vi "34970_CRISTALIZADOR_0 Module.vi"(5 "Agilent 34970A":bool=TRUE, 7 "Command":T1, 8 "error in (no error)":errorcluster, 10 "Canales":cluster{"CH PT100":string[], "CH TcK":string[]}={"CH PT100"=["201", "202", "205", "210"], "CH TcK"=["208"]}, 11 "VISA Agilent 34970A":refnum<visa-resource-name>="COM42") -> (0 "error out":errorcluster, 2 "TcK":dbl[](array[numeric]), 3 "PT100":dbl[](array[numeric]))   [LabVIEW 2017]
uses:
  34970_CRISTALIZADOR Module.ctl
  <instrlib>/Agilent 34970/Agilent 34970.lvlib
panel:
  # "Input Data"
  # "Output Data"
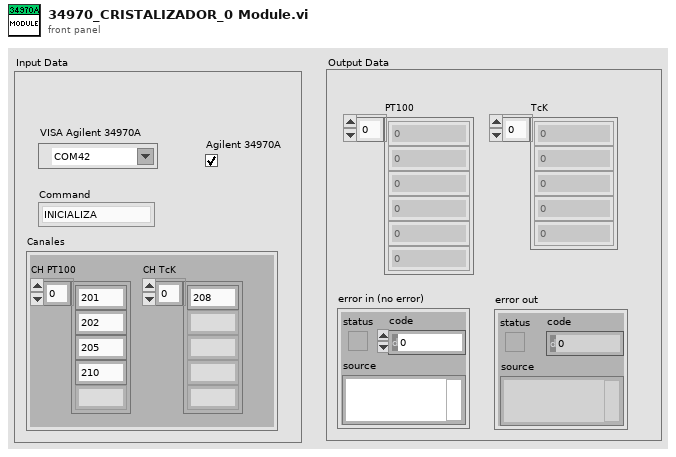
[diagram p1: front panel]
types:
  T1 = typedef "34970_CRISTALIZADOR Module.ctl" = enum16{"INICIALIZA", "CONFIGURA CANALES", "LECTURA PT100", "LECTURA TERMOPAR", "LECTURA VOLTAJE", "LECTURA CORRIENTE", "SHUTDOWN"}
  T2 = cluster{"Timeout Value (10000)":u32, "Baud Rate (57600)":enum16{"1200", "2400", "4800", "9600", "19200", "38400", "57600", "115200"}, "Flow Control (1:XON/XOFF)":enum16{"None", "XON / XOFF", "RTS / CTS", "DTR / DSR"}}
  T3 = enum16{"Thermocouple", "Thermistor", "RTD", "4-Wire RTD", "Default (Last)"}
  T4 = enum16{"B", "E", "J", "K", "N", "R", "S", "T", "Default (Last)"}
  T5 = enum16{"100 mV", "1 V", "10 V", "100 V", "300 V", "Auto", "Minimum", "Maximum"}
  T6 = enum16{"4 1/2", "5 1/2", "6 1/2", "Least", "Highest", "Default"}
  T7 = enum16{"10 mA", "100 mA", "1 A", "Auto", "Minimum", "Maximum"}
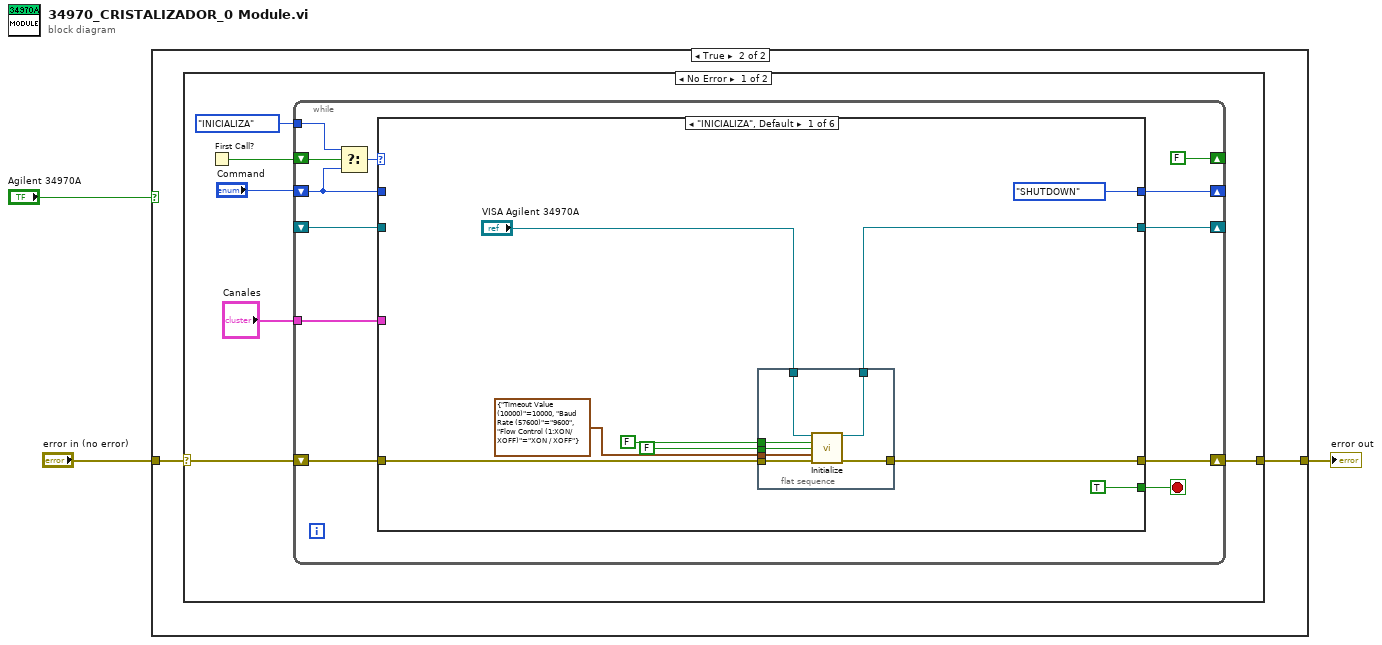
[diagram p0: block diagram]
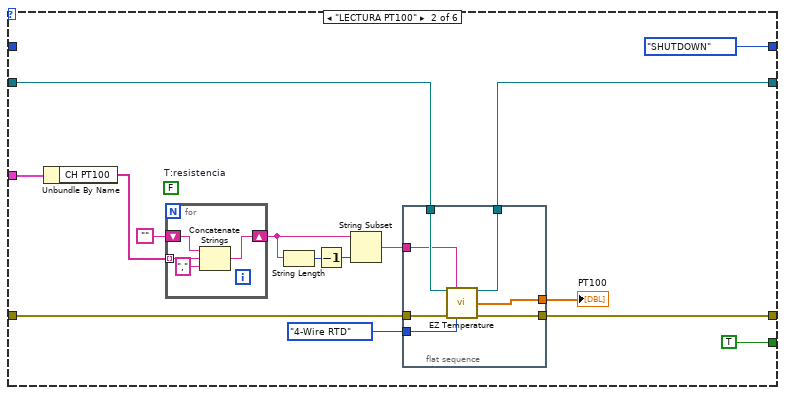
[diagram p3: hidden frame]
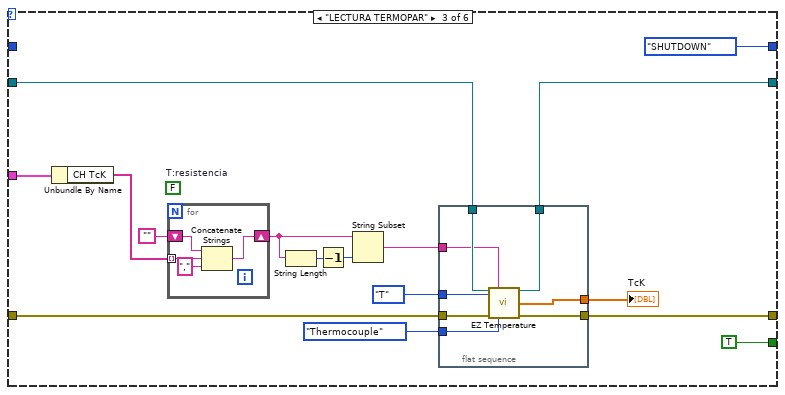
[diagram p4: hidden frame]
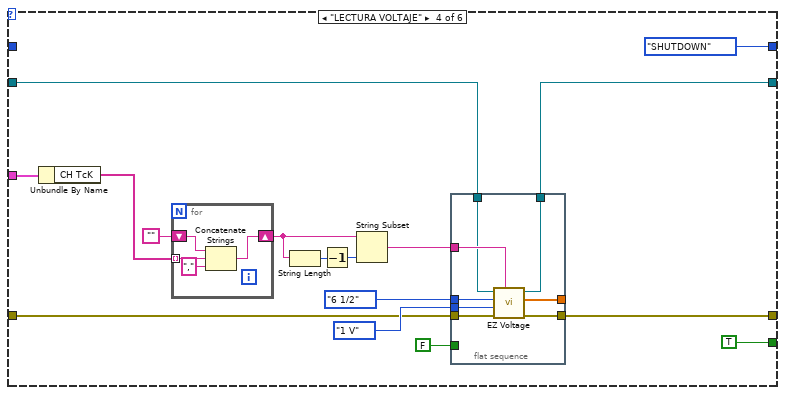
[diagram p5: hidden frame]
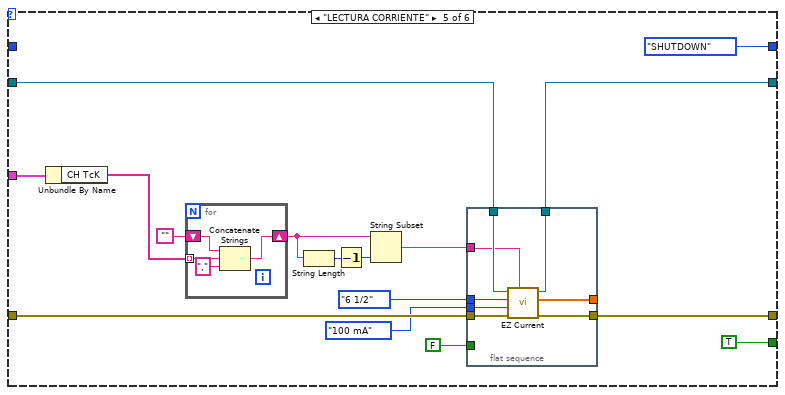
[diagram p6: hidden frame]
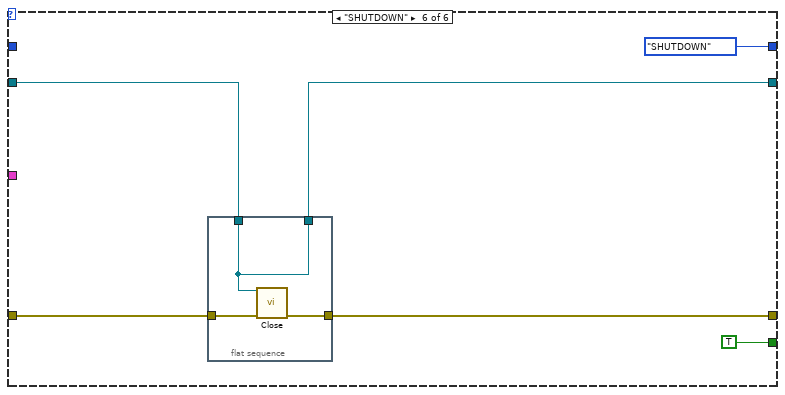
[diagram p7: hidden frame]
diagram:
  n1 = case shown="True" "Agilent 34970A" {
    tunnel: "error in (no error)" -> [w4 w6]
    tunnel: [w4 w5] -> w2
    frame False {
    }
    frame True {
      n2 = case shown="No Error" w6 {
        selector: w6 -> [w10 w160]
        tunnel: [w9 w160] -> w5
        frame No Error {
          n3 = First Call?() -> (First Call?: T/F=w12:bool)
          n4 = while {
            shift-right: [w18] -> _
            shift-left: "Command" -> [w19]
            shift-right: [w17] -> w9
            shift-left: w10 -> [w21]
            shift-right: [FALSE ("First Call?: T/F")] -> _
            shift-left: w12 -> [w24]
            tunnel: 34970_CRISTALIZADOR_Module."INICIALIZA" ("t") -> [w23]
            shift-right: [w15] -> _
            shift-left: _ -> [w16]
            tunnel: "Canales" -> [w13]
            stop <- w22 stop-if-true
            n5 = Select(t=w23, s=w24, f=w19) -> (s? t:f=w14:T1)
            n6 = case shown="\"INICIALIZA\", Default" w14 {
              tunnel: [TRUE TRUE TRUE TRUE TRUE TRUE] -> w22
              tunnel: w21 -> [w30 w52 w79 w98 w128 w156]
              tunnel: w19 -> [_ _ _ _ _ _]
              tunnel: [34970_CRISTALIZADOR_Module."SHUTDOWN" ("t") 34970_CRISTALIZADOR_Module."SHUTDOWN" ("t") 34970_CRISTALIZADOR_Module."SHUTDOWN" ("t") 34970_CRISTALIZADOR_Module."SHUTDOWN" ("t") 34970_CRISTALIZADOR_Module."SHUTDOWN" ("t") 34970_CRISTALIZADOR_Module."SHUTDOWN" ("t")] -> w18
              tunnel: [w29 w46 w73 w107 w135 w155] -> w17
              tunnel: w16 -> [_ w53 w80 w97 w127 w152]
              tunnel: [w28 w45 w72 w108 w136 w151] -> w15
              tunnel: w13 -> [_ w43 w71 w96 w124 _]
              frame "INICIALIZA", Default {
                n7 = flat-sequence {
                  tunnel: "VISA Agilent 34970A" -> [w39]
                  tunnel: w30 -> [w38]
                  tunnel: [w37] -> w29
                  tunnel: [w40] -> w28
                  tunnel: T2 {"Timeout Value (10000)"=10000, "Baud Rate (57600)"=enum."9600", "Flow Control (1:XON/XOFF)"=enum."XON / XOFF"} ("Serial Port Configuration") -> [w36]
                  tunnel: FALSE ("Reset (T: Reset)") -> [w35]
                  tunnel: FALSE ("ID Query (T: Check)") -> [w34]
                  frame #0 {
                    n8 = call <instrlib>:"Initialize.vi"("VISA Resource Name"=w39, "ID Query (T: Check)"=w34, "Reset (T: Reset)"=w35, "Serial Port Configuration"=w36, "error in (no error)"=w38) -> ("VISA Resource Name Out"=w40:refnum<visa-resource-name>, "error out"=w37:errorcluster)  [unwired: 9 in]
                  }
                }
              }
              frame "LECTURA PT100" {
                (unwired) FALSE  # T:resistencia
                n9 = Unbundle By Name(w43) -> ("CH PT100"=w42:string[])
                n10 = for {
                  tunnel: w42 -> [w65] mode=indexing
                  shift-right: [w64] -> w51
                  shift-left: "" -> [w66]
                  n11 = Concatenate Strings(w66, w65, "," ("string")) -> (w64:string)
                }
                n12 = String Length(string=w51) -> (length=w49:i32)
                n13 = Decrement(x=w49) -> (x-1=w50:i32)
                n14 = String Subset(string=w51, length (rest)=w50) -> (substring=w47:string)  [unwired: 1 in]
                n15 = flat-sequence {
                  tunnel: w53 -> [w62]
                  tunnel: w52 -> [w58]
                  tunnel: w47 -> [w56]
                  tunnel: [w60] -> w46
                  tunnel: [w61] -> w45
                  tunnel: [w59] -> w44
                  tunnel: T3."4-Wire RTD" ("Transducer Type (4:Def-Last)") -> [w57]
                  frame #0 {
                    n16 = call <instrlib>:"EZ Temperature.vi"("VISA Resource Name"=w62, "Scan List (empty)"=w56, "error in (no error)"=w58, "Transducer Type (4:Def-Last)"=w57) -> ("VISA Resource Name Out"=w61:refnum<visa-resource-name>, "Output Array"=w59:dbl[], "error out"=w60:errorcluster)  [unwired: 9 in]
                  }
                }
                "PT100" <- w44
              }
              frame "LECTURA TERMOPAR" {
                (unwired) FALSE  # T:resistencia
                n17 = Unbundle By Name(w71) -> ("CH TcK"=w70:string[])
                n18 = for {
                  tunnel: w70 -> [w93] mode=indexing
                  shift-right: [w92] -> w78
                  shift-left: "" -> [w94]
                  n19 = Concatenate Strings(w94, w93, "," ("string")) -> (w92:string)
                }
                n20 = String Length(string=w78) -> (length=w76:i32)
                n21 = Decrement(x=w76) -> (x-1=w77:i32)
                n22 = String Subset(string=w78, length (rest)=w77) -> (substring=w74:string)  [unwired: 1 in]
                n23 = flat-sequence {
                  tunnel: w80 -> [w90]
                  tunnel: w79 -> [w86]
                  tunnel: w74 -> [w84]
                  tunnel: [w88] -> w73
                  tunnel: [w89] -> w72
                  tunnel: [w87] -> w68
                  tunnel: T3."Thermocouple" ("Transducer Type (4:Def-Last)") -> [w85]
                  tunnel: T4."T" ("Thermocouple Type (8:Def-Last)") -> [w83]
                  frame #0 {
                    n24 = call <instrlib>:"EZ Temperature.vi"("VISA Resource Name"=w90, "Scan List (empty)"=w84, "Thermocouple Type (8:Def-Last)"=w83, "error in (no error)"=w86, "Transducer Type (4:Def-Last)"=w85) -> ("VISA Resource Name Out"=w89:refnum<visa-resource-name>, "Output Array"=w87:dbl[], "error out"=w88:errorcluster)  [unwired: 8 in]
                  }
                }
                "TcK" <- w68
              }
              frame "LECTURA VOLTAJE" {
                n25 = Unbundle By Name(w96) -> ("CH TcK"=w95:string[])
                n26 = for {
                  tunnel: w95 -> [w121] mode=indexing
                  shift-right: [w120] -> w106
                  shift-left: "" -> [w122]
                  n27 = Concatenate Strings(w122, w121, "," ("string")) -> (w120:string)
                }
                n28 = String Length(string=w106) -> (length=w104:i32)
                n29 = Decrement(x=w104) -> (x-1=w105:i32)
                n30 = String Subset(string=w106, length (rest)=w105) -> (substring=w99:string)  [unwired: 1 in]
                n31 = flat-sequence {
                  tunnel: [w111] -> w108
                  tunnel: [w115] -> w107
                  tunnel: FALSE ("AC/DC (F:DC)") -> [_]
                  tunnel: T6."6 1/2" ("Resolution (5:Default)") -> [w112]
                  tunnel: T5."1 V" ("Range (5:Auto)") -> [w113]
                  tunnel: w99 -> [w118]
                  tunnel: w98 -> [w114]
                  tunnel: w97 -> [w117]
                  tunnel: [w116] -> _
                  frame #0 {
                    n32 = call <instrlib>:"EZ Voltage.vi"("Scan List (empty)"=w118, "error in (no error)"=w114, "Range (5:Auto)"=w113, "Resolution (5:Default)"=w112, "VISA Resource Name"=w117) -> ("error out"=w115:errorcluster, "Output Array"=w116:dbl[], "VISA Resource Name Out"=w111:refnum<visa-resource-name>)  [unwired: 4 in]
                  }
                }
              }
              frame "LECTURA CORRIENTE" {
                n33 = Unbundle By Name(w124) -> ("CH TcK"=w123:string[])
                n34 = for {
                  tunnel: w123 -> [w149] mode=indexing
                  shift-right: [w148] -> w134
                  shift-left: "" -> [w150]
                  n35 = Concatenate Strings(w150, w149, "," ("string")) -> (w148:string)
                }
                n36 = String Length(string=w134) -> (length=w132:i32)
                n37 = Decrement(x=w132) -> (x-1=w133:i32)
                n38 = String Subset(string=w134, length (rest)=w133) -> (substring=w129:string)  [unwired: 1 in]
                n39 = flat-sequence {
                  tunnel: [w145] -> w136
                  tunnel: [w143] -> w135
                  tunnel: FALSE ("AC/DC (F:DC)") -> [_]
                  tunnel: w129 -> [w139]
                  tunnel: w128 -> [w144]
                  tunnel: w127 -> [w146]
                  tunnel: T6."6 1/2" ("Resolution (3:Least)") -> [w141]
                  tunnel: T7."100 mA" ("Range (3:Auto)") -> [w140]
                  tunnel: [w142] -> _
                  frame #0 {
                    n40 = call <instrlib>:"EZ Current.vi"("Scan List (empty)"=w139, "error in (no error)"=w144, "Range (3:Auto)"=w140, "Resolution (3:Least)"=w141, "VISA Resource Name"=w146) -> ("error out"=w143:errorcluster, "Output Array"=w142:dbl[], "VISA Resource Name Out"=w145:refnum<visa-resource-name>)  [unwired: 4 in]
                  }
                }
              }
              frame "SHUTDOWN" {
                n41 = flat-sequence {
                  tunnel: w156 -> [w158]
                  tunnel: [w157] -> w155
                  tunnel: [w159] -> w151
                  tunnel: w152 -> [w159]
                  frame #0 {
                    n42 = call <instrlib>:"Close.vi"("VISA Resource Name"=w159, "error in (no error)"=w158) -> ("error out"=w157:errorcluster)  [unwired: 13 in]
                  }
                }
              }
            }
          }
        }
        frame Error {
        }
      }
    }
  }
  "error out" <- w2
